vi "Select ch str (SubVI).vi"(10 "字符串":string, 11 "队列输入":refnum<queue>) -> ()   [LabVIEW 2019, in "Take Seq.lvlib"]
uses:
  Take Seq.lvlib
  config.ctl
  lib/QDInstrument.dll
  KE7001.LLB/Keith 7001 Open/Close Chan.vi
  SubVI.lvlib
panel:
  # "(真是通道1，假是通道2)"
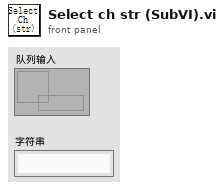
[diagram p1: front panel]
types:
  T1 = typedef "config.ctl" = cluster{"initialize":string, "6221":cluster{"6221 Resource":refnum<visa-resource-name>, "Delta status":bool}, "7001":cluster{"Ch":bool}, "SR830+6221":cluster{"source":u16, "阻抗":dbl, "量程入 4":i32, "量程入 3":i32, "量程入 2":i32, "量程入 1":i32, "电流":dbl, "SR830 2":bool, "SR830 3":bool, "SR830 4":bool, "SR830 1":bool, "VISA 1":refnum<visa-resource-name>, "VISA 2":refnum<visa-resource-name>, "VISA 3":refnum<visa-resource-name>, "VISA 4":refnum<visa-resource-name>, "量程":enum16{"量程每次测量会判定", "量程不变为设定值"}}, "2400":cluster{"2400":bool, "VISA":refnum<visa-resource-name>}, "ch":cluster{"ch str":string, "ch1":bool, "ch2":bool, "布尔":bool}, "quantum design":refnum<k24>, "error":bool, "数据文件路径":path, "log":cluster{"log路径":path, "log interval":dbl}}
  T2 = cluster{"slot/memory":i16, "channel/row":i16, "column":i16, bool, bool}[]
  T3 = cluster{"error":bool, "code":i32, "source":string}
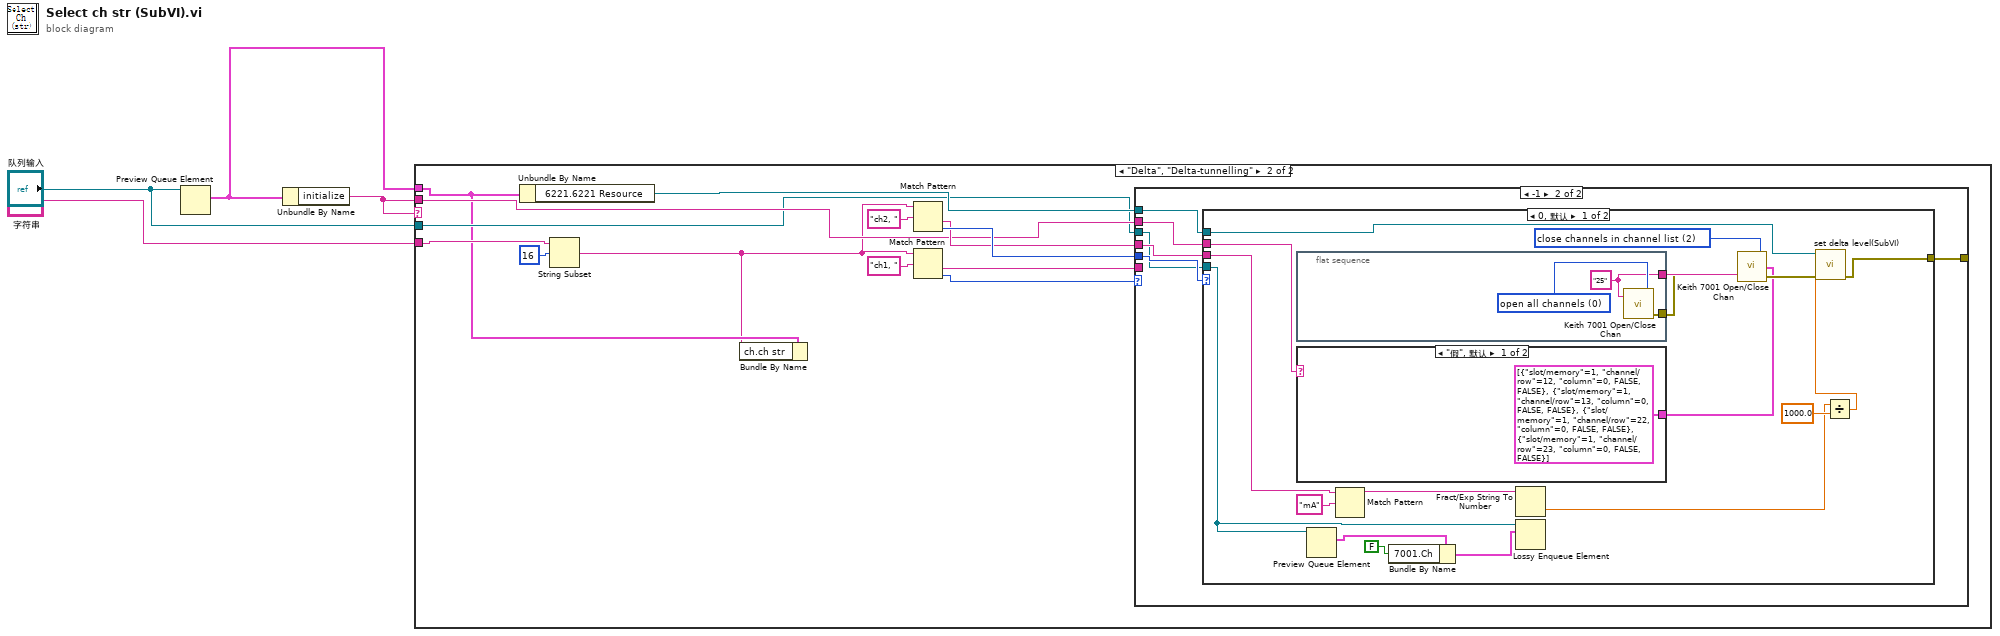
[diagram p0: block diagram]
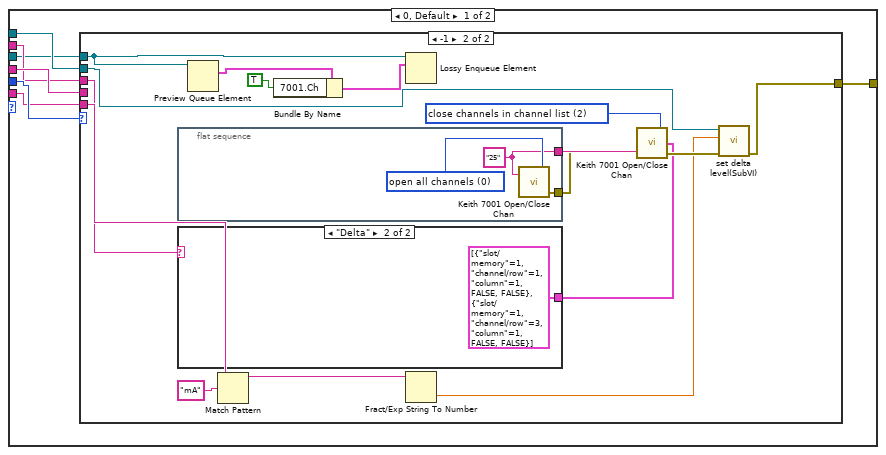
[diagram p3: hidden frame]
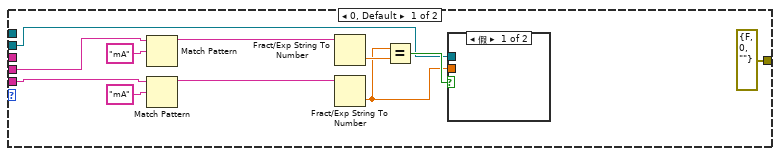
[diagram p4: hidden frame]
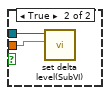
[diagram p5: hidden frame]
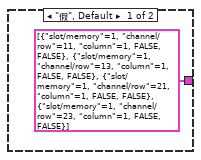
[diagram p6: hidden frame]
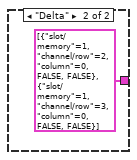
[diagram p7: hidden frame]
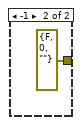
[diagram p8: hidden frame]
diagram:
  n1 = Preview Queue Element(queue="队列输入") -> (element=w3:T1)  [unwired: 2 in, 3 out]
  n2 = Unbundle By Name(w3) -> ("initialize"=w2:string)
  n3 = case shown="\"Delta\", \"Delta-tunnelling\"" w2 {
    tunnel: "字符串" -> [_ w16]
    tunnel: w2 -> [_ w9]
    tunnel: w3 -> [_ w6]
    tunnel: "队列输入" -> [_ w7]
    frame "假", Default {
    }
    frame "Delta", "Delta-tunnelling" {
      n4 = Unbundle By Name(w6) -> ("6221.6221 Resource"=w8:refnum<visa-resource-name>)
      n5 = String Subset(string=w16, offset (0)=16 ("偏移量(0)")) -> (substring=w5:string)  [unwired: 1 in]
      n6 = Bundle By Name(cluster=w6, "ch.ch str"=w5) -> ()  [unwired: 1 out]
      n7 = Match Pattern(string=w5, regular expression="ch2, " ("正则表达式")) -> (after substring=w10:string, offset past match=w12:i32)  [unwired: 1 in, 2 out]
      n8 = Match Pattern(string=w5, regular expression="ch1, " ("正则表达式")) -> (after substring=w11:string, offset past match=w14:i32)  [unwired: 1 in, 2 out]
      n9 = case shown="-1" w14 {
        tunnel: w12 -> [w24 w64]
        tunnel: w8 -> [w23 w62]
        tunnel: [w22 w61] -> _
        tunnel: w11 -> [w21 _]
        tunnel: w10 -> [w20 w63]
        tunnel: w9 -> [w19 w60]
        tunnel: w7 -> [w18 w59]
        frame 0, Default {
          n10 = case shown="-1" w24 {
            tunnel: [errorcluster {"status"=FALSE, "code"=0, "source"=""} ("错误输出") w49] -> w22
            tunnel: w23 -> [w25 w48]
            tunnel: w21 -> [w29 w47]
            tunnel: w20 -> [w28 _]
            tunnel: w19 -> [_ w42]
            tunnel: w18 -> [_ w38]
            frame 0, Default {
              n11 = Match Pattern(string=w28, regular expression="mA" ("正则表达式")) -> (before substring=w32:string)  [unwired: 1 in, 3 out]
              n12 = Match Pattern(string=w29, regular expression="mA" ("正则表达式")) -> (before substring=w31:string)  [unwired: 1 in, 3 out]
              n13 = Fract/Exp String To Number(string=w32) -> (number=w30:dbl)  [unwired: 3 in, 1 out]
              n14 = Fract/Exp String To Number(string=w31) -> (number=w26:dbl)  [unwired: 3 in, 1 out]
              n15 = Equal?(x=w26, y=w30) -> (x = y?=w27:bool)
              n16 = case shown="假" w27 {
                tunnel: w26 -> [_ w37]
                tunnel: w25 -> [_ w36]
                frame False {
                }
                frame True {
                  n17 = call "set delta level(SubVI).vi"("电流（A）"=w37, "VISA引用句柄输入"=w36) -> ()  [unwired: 8 in, 2 out]
                }
              }
            }
            frame -1 {
              w52 = u16 2 items=["open all channels", "open channels in channel list", "close channels in channel list"] ("open/close (open all:0)")
              n18 = flat-sequence {
                tunnel: [w57] -> w53
                tunnel: [w56] -> w50
                frame #0 {
                  w58 = u16 0 items=["open all channels", "open channels in channel list", "close channels in channel list"] ("open/close (open all:0)")
                  w57 = "25" ("GPIB address")
                  n19 = call "Keith 7001 Open/Close Chan.vi"("GPIB address"=w57, "open/close (open all:0)"=w58) -> ("error out"=w56:T3)  [unwired: 2 in]
                }
              }
              n20 = case shown="\"Delta\"" w42 {
                tunnel: [T2 [{"slot/memory"=1, "channel/row"=11, "column"=1, FALSE, FALSE}, {"slot/memory"=1, "channel/row"=13, "column"=1, FALSE, FALSE}, {"slot/memory"=1, "channel/row"=21, "column"=1, FALSE, FALSE}, {"slot/memory"=1, "channel/row"=23, "column"=1, FALSE, FALSE}] ("channel list") T2 [{"slot/memory"=1, "channel/row"=1, "column"=1, FALSE, FALSE}, {"slot/memory"=1, "channel/row"=3, "column"=1, FALSE, FALSE}] ("channel list")] -> w43
                frame "假", Default {
                }
                frame "Delta" {
                }
              }
              n21 = Preview Queue Element(queue=w38) -> (element=w39:T1)  [unwired: 2 in, 3 out]
              n22 = Match Pattern(string=w47, regular expression="mA" ("正则表达式")) -> (before substring=w44:string)  [unwired: 1 in, 3 out]
              n23 = Bundle By Name(cluster=w39, "7001.Ch"=TRUE) -> (w40:T1)
              n24 = Lossy Enqueue Element(queue=w38, element=w40) -> ()  [unwired: 1 in, 4 out]
              n25 = Fract/Exp String To Number(string=w44) -> (number=w45:dbl)  [unwired: 3 in, 1 out]
              n26 = call "Keith 7001 Open/Close Chan.vi"("GPIB address"=w53, "error in"=w50, "open/close (open all:0)"=w52, "channel list"=w43) -> ("error out"=w51:T3)
              n27 = call "set delta level(SubVI).vi"("错误输入（无错误）"=w51, "电流（A）"=w45, "VISA引用句柄输入"=w48) -> ("错误输出"=w49:errorcluster)  [unwired: 7 in, 1 out]
            }
          }
        }
        frame -1 {
          n28 = case shown="0, 默认" w64 {
            tunnel: w63 -> [w79 _]
            tunnel: w62 -> [w78 _]
            tunnel: [w75 errorcluster {"status"=FALSE, "code"=0, "source"=""} ("错误输出")] -> w61
            tunnel: w60 -> [w73 _]
            tunnel: w59 -> [w68 _]
            frame 0, Default {
              w81 = u16 2 items=["open all channels", "open channels in channel list", "close channels in channel list"] ("open/close (open all:0)")
              n29 = flat-sequence {
                tunnel: [w86] -> w82
                tunnel: [w85] -> w76
                frame #0 {
                  w87 = u16 0 items=["open all channels", "open channels in channel list", "close channels in channel list"] ("open/close (open all:0)")
                  w86 = "25" ("GPIB address")
                  n30 = call "Keith 7001 Open/Close Chan.vi"("GPIB address"=w86, "open/close (open all:0)"=w87) -> ("error out"=w85:T3)  [unwired: 2 in]
                }
              }
              n31 = case shown="\"假\", 默认" w73 {
                tunnel: [T2 [{"slot/memory"=1, "channel/row"=12, "column"=0, FALSE, FALSE}, {"slot/memory"=1, "channel/row"=13, "column"=0, FALSE, FALSE}, {"slot/memory"=1, "channel/row"=22, "column"=0, FALSE, FALSE}, {"slot/memory"=1, "channel/row"=23, "column"=0, FALSE, FALSE}] ("channel list") T2 [{"slot/memory"=1, "channel/row"=2, "column"=0, FALSE, FALSE}, {"slot/memory"=1, "channel/row"=3, "column"=0, FALSE, FALSE}] ("channel list")] -> w72
                frame "假", Default {
                }
                frame "Delta" {
                }
              }
              n32 = Preview Queue Element(queue=w68) -> (element=w69:T1)  [unwired: 2 in, 3 out]
              n33 = Match Pattern(string=w79, regular expression="mA" ("正则表达式")) -> (before substring=w74:string)  [unwired: 1 in, 3 out]
              n34 = Bundle By Name(cluster=w69, "7001.Ch"=FALSE) -> (w70:T1)
              n35 = Fract/Exp String To Number(string=w74) -> (number=w66:dbl)  [unwired: 3 in, 1 out]
              n36 = Lossy Enqueue Element(queue=w68, element=w70) -> ()  [unwired: 1 in, 4 out]
              n37 = call "Keith 7001 Open/Close Chan.vi"("GPIB address"=w82, "error in"=w76, "open/close (open all:0)"=w81, "channel list"=w72) -> ("error out"=w77:T3)
              n38 = Divide(x=w66, y=1000.0) -> (x/y=w65:dbl)
              n39 = call "set delta level(SubVI).vi"("错误输入（无错误）"=w77, "电流（A）"=w65, "VISA引用句柄输入"=w78) -> ("错误输出"=w75:errorcluster)  [unwired: 7 in, 1 out]
            }
            frame -1 {
            }
          }
        }
      }
    }
  }
